vi "Finish.vi"   [LabVIEW 2015]
doc: "This VI is called just before exiting. It is expected to close I/O refnum, save collected data, etc."
uses:
  <vilib>/Rock Robotics/WPI/Utilities/WPI_GetSetVariantRefNum.vi
  <vilib>/Rock Robotics/WPI/Ultrasonic/WPI_SonarMB1010AnalogRefNum Registry Get.vi
  <vilib>/Rock Robotics/WPI/Ultrasonic/WPI_SonarMB1010AnalogClose.vi
types:
  T1 = typedef "WPI_SonarMB1010AnalogDeviceRef.ctl" = cluster{"AIDeviceRef":T2, "Scaling factor (V/in)":dbl, "Average Bits":u8}
  T2 = typedef "WPI_AnalogChannelDevRef.ctl" = cluster{"DevStatus":errorcluster, "Analog Channel":T3}
  T3 = typedef "FPGA_AIChannel.ctl" = enum8{"AI 0", "AI 1", "AI 2", "AI 3", "AI MXP 0", "AI MXP 1", "AI MXP 2", "AI MXP 3", "Invalid"}
  T4 = typedef "WPI_ServoDeviceRef.ctl" = cluster{"DeviceStatus":errorcluster, "PWM Channel":T5, "DeadBand":T6}
  T5 = typedef "FPGA_DIOPWMChannel.ctl" = enum8{"PWM 0", "PWM 1", "PWM 2", "PWM 3", "PWM 4", "PWM 5", "PWM 6", "PWM 7", "PWM 8", "PWM 9", "PWM MXP 0", "PWM MXP 1", "PWM MXP 2", "PWM MXP 3", "PWM MXP 4", "PWM MXP 5", "PWM MXP 6", "PWM MXP 7", "PWM MXP 8", "PWM MXP 9", "Invalid"}
  T6 = typedef "WPI_PWMDeadband.ctl" = cluster{"Name":string, "maxPositivePwm":i32, "minPositivePwm":i32, "centerPwm":i32, "maxNegativePwm":i32, "minNegativePwm":i32, "angularRange":u16}
  T7 = typedef "WPI_MotorControlDeviceRef.ctl" = cluster{"DeviceStatus":errorcluster, "Type":T8, "PWM":cluster{"PWM Channel":T5, "DeadBand":T6}, "CAN":cluster{"Device Number":u8, "Control Mode":T9, "Semaphore":T10, "Max Vout":dbl, "TalonSRX Control Mode":T11}, "Invert":bool}
  T8 = typedef "WPI_MotorControlType.ctl" = enum16{"PWM", "CAN", "CANTalonSRX"}
  T9 = typedef "WPI_CANJaguar_ControlMode.ctl" = enum8{"Percent VBus", "Current", "Speed", "Position", "Voltage"}
  T10 = typedef "Semaphore RefNum" = refnum<k1>
  T11 = typedef "WPI_CANTalonSRX_APIControlMode.ctl" = enum8{"Percent VBus", "Speed", "Position", "Slave", "Unchanged / Invalid", "Voltage Compensation", "Current", "Motion Profile"}
  T12 = typedef "WPI_SolenoidDevRef.ctl" = cluster{"DevStatus":errorcluster, "Pneumatics Control Module":u8, "Forward Solenoid Channel":T13, "Reverse Solenoid Channel":T13}
  T13 = typedef "WPI_SolenoidChannel.ctl" = enum8{"Solenoid 0", "Solenoid 1", "Solenoid 2", "Solenoid 3", "Solenoid 4", "Solenoid 5", "Solenoid 6", "Solenoid 7", "Invalid"}
  T14 = typedef "WPI_JoystickDevRef.ctl" = cluster{"Device":T15}
  T15 = typedef "WPI_JoystickDeviceEnum.ctl" = enum16{"USB 0", "USB 1", "USB 2", "USB 3", "USB 4", "USB 5"}
  T16 = typedef "WPI_PotentiometerDevRef.ctl" = cluster{"DevStatus":errorcluster, "Analog Channel":T3, "Invert Output":bool}
  T17 = typedef "WPI_GyroDevRef.ctl" = cluster{"DevStatus":errorcluster, "Analog Channel":T3, "Offset":dbl, "Gain (VoltsPerDegree/Second)":dbl, "Gyro Type":enum16{"Analog", "XRS450"}, "Handle":i32, "SPI Bus":T18, "Device Found":bool, "Sample Rate":dbl, "Calibrate On Open":bool}
  T18 = typedef "spi_bus.ctl" = enum16{"SPI On-Board, CS0", "SPI On-Board, CS1", "SPI On-Board, CS2", "SPI On-Board, CS3", "SPI MXP", "Invalid"}
  T19 = typedef "WPI_EncoderDevRef.ctl" = cluster{"DevStatus":errorcluster, "EncoderIndex":T20, "CounterIndex":T21, "DistancePerCount":dbl, "Decoding Type":T22}
  T20 = typedef "FPGA_EncoderIdx.ctl" = enum8{"Enc 0", "Enc 1", "Enc 2", "Enc 3", "Enc 4", "Enc 5", "Enc 6", "Enc 7", "Invalid"}
  T21 = typedef "FPGA_CounterCtrSystemIndex.ctl" = enum8{"Ctr 0", "Ctr 1", "Ctr 2", "Ctr 3", "Ctr 4", "Ctr 5", "Ctr 6", "Ctr 7", "Invalid"}
  T22 = typedef "WPI_EncoderType.ctl" = enum16{"1x", "2x", "4x"}
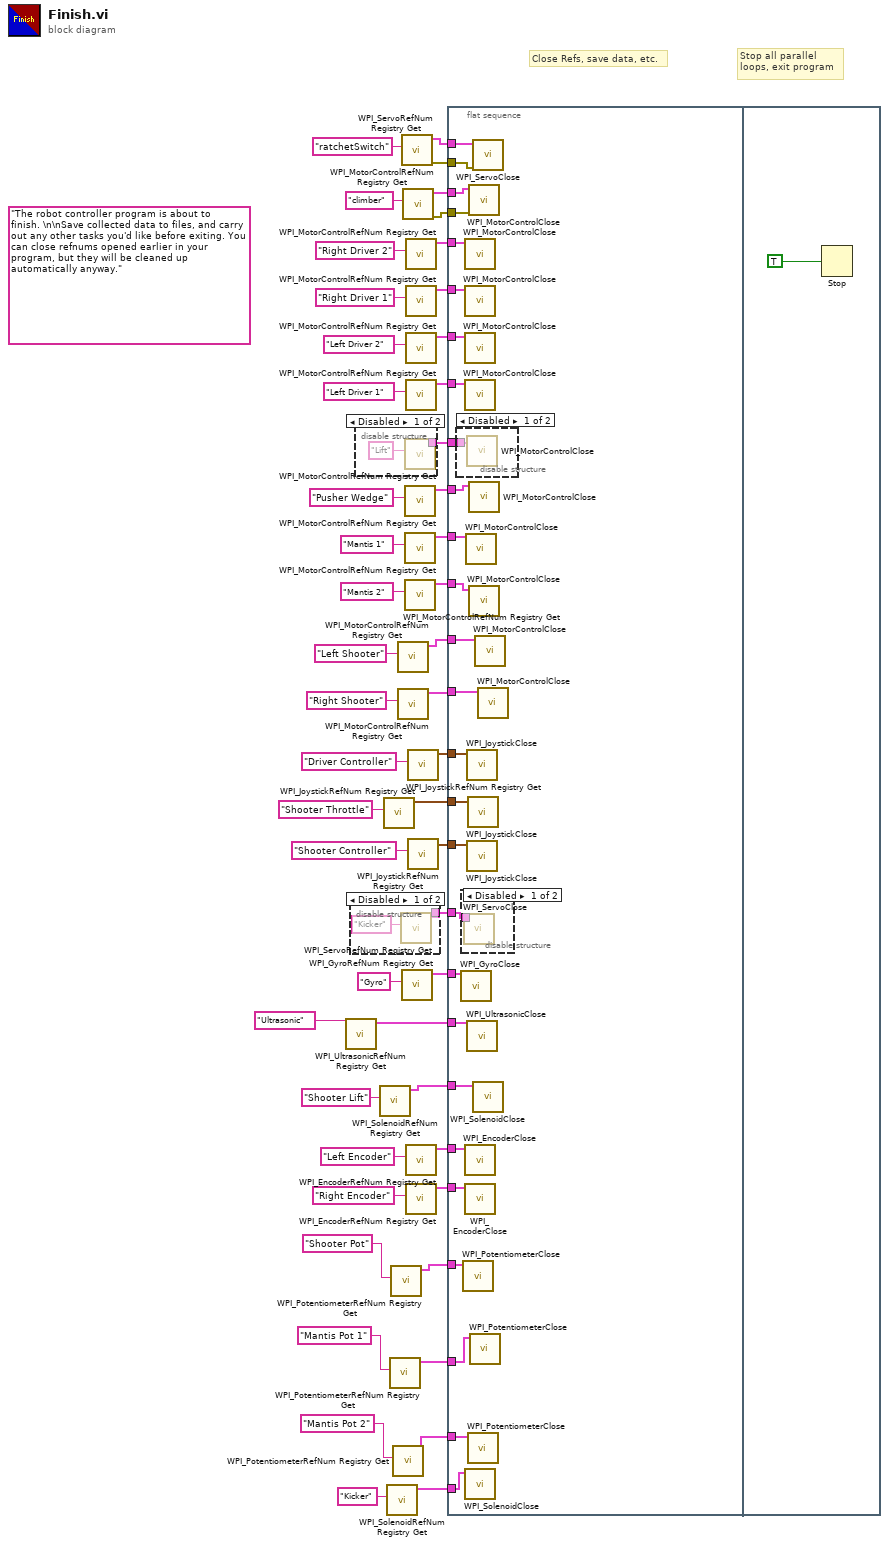
[diagram p0: block diagram]
diagram:
  (unwired) "The robot controller program is about to finish. \n\nSave collected data to files, and carry out any other tasks you'd like before exiting. You can close refnums opened earlier in your program, but they will be cleaned up automatically anyway."
  # "Stop all parallel\nloops, exit program"
  # "Close Refs, save data, etc."
  n1 = call-poly <vilib>:"WPI_UltrasonicRefNum Registry Get.vi"("refnum name"="Ultrasonic") -> ("SonarMB1010AnalogDevRef"=w20:T1)  [unwired: 9 in, 1 out]
  n2 = disable-structure shown="Disabled" {
    disable-tunnel: [w52 _] -> w21
    frame Disabled {
      n3 = call <vilib>:"WPI_ServoRefNum Registry Get.vi"("refnum name"="Kicker") -> ("ServoDeviceRef"=w52:T4)  [unwired: 9 in, 1 out]
    }
    frame Enabled {
    }
  }
  n4 = disable-structure shown="Disabled" {
    disable-tunnel: [w53 _] -> w26
    frame Disabled {
      n5 = call <vilib>:"WPI_MotorControlRefNum Registry Get.vi"("refnum name"="Lift") -> ("MotorControlDevRef"=w53:T7)  [unwired: 9 in, 1 out]
    }
    frame Enabled {
    }
  }
  n6 = call <vilib>:"WPI_SolenoidRefNum Registry Get.vi"("refnum name"="Shooter Lift") -> ("SolenoidDevRef"=w10:T12)  [unwired: 9 in, 1 out]
  n7 = call <vilib>:"WPI_JoystickRefNum Registry Get.vi"("refnum name"="Shooter Throttle") -> ("JoystickDevRef"=w11:T14)  [unwired: 9 in, 1 out]
  n8 = call <vilib>:"WPI_SolenoidRefNum Registry Get.vi"("refnum name"="Kicker") -> ("SolenoidDevRef"=w8:T12)  [unwired: 9 in, 1 out]
  n9 = call <vilib>:"WPI_PotentiometerRefNum Registry Get.vi"("refnum name"="Mantis Pot 1") -> ("PotDevRef"=w14:T16)  [unwired: 9 in, 1 out]
  n10 = call <vilib>:"WPI_PotentiometerRefNum Registry Get.vi"("refnum name"="Shooter Pot") -> ("PotDevRef"=w13:T16)  [unwired: 9 in, 1 out]
  n11 = call <vilib>:"WPI_PotentiometerRefNum Registry Get.vi"("refnum name"="Mantis Pot 2") -> ("PotDevRef"=w15:T16)  [unwired: 9 in, 1 out]
  n12 = call <vilib>:"WPI_MotorControlRefNum Registry Get.vi"("refnum name"="Left Shooter") -> ("MotorControlDevRef"=w23:T7)  [unwired: 9 in, 1 out]
  n13 = call <vilib>:"WPI_MotorControlRefNum Registry Get.vi"("refnum name"="Right Shooter") -> ("MotorControlDevRef"=w22:T7)  [unwired: 9 in, 1 out]
  n14 = call <vilib>:"WPI_ServoRefNum Registry Get.vi"("refnum name"="ratchetSwitch") -> ("error out"=w5:errorcluster, "ServoDeviceRef"=w6:T4)  [unwired: 9 in]
  n15 = call <vilib>:"WPI_GyroRefNum Registry Get.vi"("refnum name"="Gyro") -> ("GyroDevRef"=w33:T17)  [unwired: 9 in, 1 out]
  n16 = call <vilib>:"WPI_MotorControlRefNum Registry Get.vi"("refnum name"="climber") -> ("error out"=w3:errorcluster, "MotorControlDevRef"=w4:T7)  [unwired: 9 in]
  n17 = call <vilib>:"WPI_MotorControlRefNum Registry Get.vi"("refnum name"="Pusher Wedge") -> ("MotorControlDevRef"=w27:T7)  [unwired: 9 in, 1 out]
  n18 = call <vilib>:"WPI_MotorControlRefNum Registry Get.vi"("refnum name"="Mantis 1") -> ("MotorControlDevRef"=w28:T7)  [unwired: 9 in, 1 out]
  n19 = call <vilib>:"WPI_MotorControlRefNum Registry Get.vi"("refnum name"="Mantis 2") -> ("MotorControlDevRef"=w29:T7)  [unwired: 9 in, 1 out]
  n20 = call <vilib>:"WPI_MotorControlRefNum Registry Get.vi"("refnum name"="Right Driver 2") -> ("MotorControlDevRef"=w46:T7)  [unwired: 9 in, 1 out]
  n21 = call <vilib>:"WPI_MotorControlRefNum Registry Get.vi"("refnum name"="Right Driver 1") -> ("MotorControlDevRef"=w45:T7)  [unwired: 9 in, 1 out]
  n22 = call <vilib>:"WPI_MotorControlRefNum Registry Get.vi"("refnum name"="Left Driver 2") -> ("MotorControlDevRef"=w44:T7)  [unwired: 9 in, 1 out]
  n23 = call <vilib>:"WPI_MotorControlRefNum Registry Get.vi"("refnum name"="Left Driver 1") -> ("MotorControlDevRef"=w43:T7)  [unwired: 9 in, 1 out]
  n24 = call <vilib>:"WPI_EncoderRefNum Registry Get.vi"("refnum name"="Left Encoder") -> ("EncoderDevRef"=w40:T19)  [unwired: 9 in, 1 out]
  n25 = call <vilib>:"WPI_EncoderRefNum Registry Get.vi"("refnum name"="Right Encoder") -> ("EncoderDevRef"=w39:T19)  [unwired: 9 in, 1 out]
  n26 = call <vilib>:"WPI_JoystickRefNum Registry Get.vi"("refnum name"="Driver Controller") -> ("JoystickDevRef"=w38:T14)  [unwired: 9 in, 1 out]
  n27 = call <vilib>:"WPI_JoystickRefNum Registry Get.vi"("refnum name"="Shooter Controller") -> ("JoystickDevRef"=w37:T14)  [unwired: 9 in, 1 out]
  n28 = flat-sequence {
    tunnel: w46 -> [w81]
    tunnel: w45 -> [w80]
    tunnel: w44 -> [w79]
    tunnel: w43 -> [w78]
    tunnel: w40 -> [w77]
    tunnel: w39 -> [w76]
    tunnel: w38 -> [w75]
    tunnel: w37 -> [w74]
    tunnel: w33 -> [w73]
    tunnel: w29 -> [w72]
    tunnel: w28 -> [w71]
    tunnel: w27 -> [w70]
    tunnel: w26 -> [w69]
    tunnel: w23 -> [w68]
    tunnel: w22 -> [w67]
    tunnel: w21 -> [w66]
    tunnel: w20 -> [w65]
    tunnel: w15 -> [w64]
    tunnel: w14 -> [w63]
    tunnel: w13 -> [w62]
    tunnel: w11 -> [w61]
    tunnel: w10 -> [w60]
    tunnel: w8 -> [w59]
    tunnel: w6 -> [w58]
    tunnel: w5 -> [w57]
    tunnel: w4 -> [w56]
    tunnel: w3 -> [w55]
    frame #0 {
      n29 = disable-structure shown="Disabled" {
        disable-tunnel: w69 -> [w83 _]
        frame Disabled {
          n30 = call <vilib>:"WPI_MotorControlClose.vi"("MotorControlDevRef"=w83) -> ()  [unwired: 10 in, 1 out]
        }
        frame Enabled {
        }
      }
      n31 = call <vilib>:"WPI_GyroClose.vi"("GyroDevRef"=w73) -> ()  [unwired: 10 in, 1 out]
      n32 = disable-structure shown="Disabled" {
        disable-tunnel: w66 -> [w82 _]
        frame Disabled {
          n33 = call <vilib>:"WPI_ServoClose.vi"("ServoDeviceRef"=w82) -> ()  [unwired: 10 in, 1 out]
        }
        frame Enabled {
        }
      }
      n34 = call <vilib>:"WPI_PotentiometerClose.vi"("PotDevRef"=w62) -> ()  [unwired: 10 in, 1 out]
      n35 = call <vilib>:"WPI_MotorControlClose.vi"("MotorControlDevRef"=w81) -> ()  [unwired: 10 in, 1 out]
      n36 = call <vilib>:"WPI_MotorControlClose.vi"("MotorControlDevRef"=w80) -> ()  [unwired: 10 in, 1 out]
      n37 = call <vilib>:"WPI_MotorControlClose.vi"("MotorControlDevRef"=w79) -> ()  [unwired: 10 in, 1 out]
      n38 = call <vilib>:"WPI_MotorControlClose.vi"("MotorControlDevRef"=w78) -> ()  [unwired: 10 in, 1 out]
      n39 = call <vilib>:"WPI_EncoderClose.vi"("EncoderDevRef"=w77) -> ()  [unwired: 10 in, 1 out]
      n40 = call <vilib>:"WPI_EncoderClose.vi"("EncoderDevRef"=w76) -> ()  [unwired: 10 in, 1 out]
      n41 = call <vilib>:"WPI_SolenoidClose.vi"("SolenoidDevRef"=w59) -> ()  [unwired: 10 in, 1 out]
      n42 = call <vilib>:"WPI_MotorControlClose.vi"("MotorControlDevRef"=w71) -> ()  [unwired: 10 in, 1 out]
      n43 = call <vilib>:"WPI_JoystickClose.vi"("JoystickDevRef"=w75) -> ()  [unwired: 11 in]
      n44 = call <vilib>:"WPI_JoystickClose.vi"("JoystickDevRef"=w74) -> ()  [unwired: 11 in]
      n45 = call-poly <vilib>:"WPI_UltrasonicClose.vi"("SonarMB1010AnalogDevRef"=w65) -> ()  [unwired: 10 in, 1 out]
      n46 = call <vilib>:"WPI_JoystickClose.vi"("JoystickDevRef"=w61) -> ()  [unwired: 11 in]
      n47 = call <vilib>:"WPI_PotentiometerClose.vi"("PotDevRef"=w64) -> ()  [unwired: 10 in, 1 out]
      n48 = call <vilib>:"WPI_MotorControlClose.vi"("error in (no error)"=w55, "MotorControlDevRef"=w56) -> ()  [unwired: 9 in, 1 out]
      n49 = call <vilib>:"WPI_MotorControlClose.vi"("MotorControlDevRef"=w70) -> ()  [unwired: 10 in, 1 out]
      n50 = call <vilib>:"WPI_MotorControlClose.vi"("MotorControlDevRef"=w72) -> ()  [unwired: 10 in, 1 out]
      n51 = call <vilib>:"WPI_PotentiometerClose.vi"("PotDevRef"=w63) -> ()  [unwired: 10 in, 1 out]
      n52 = call <vilib>:"WPI_ServoClose.vi"("error in (no error)"=w57, "ServoDeviceRef"=w58) -> ()  [unwired: 9 in, 1 out]
      n53 = call <vilib>:"WPI_SolenoidClose.vi"("SolenoidDevRef"=w60) -> ()  [unwired: 10 in, 1 out]
      n54 = call <vilib>:"WPI_MotorControlClose.vi"("MotorControlDevRef"=w68) -> ()  [unwired: 10 in, 1 out]
      n55 = call <vilib>:"WPI_MotorControlClose.vi"("MotorControlDevRef"=w67) -> ()  [unwired: 10 in, 1 out]
    }
    frame #1 {
      n56 = Stop(stop? (T)=TRUE ("Quit")) -> ()
    }
  }
